vi "RTShutdown.vi"(0 "FPGA VI Reference In":refnum<k20>, 3 "error in (no error)":errorcluster) -> (10 "error out":errorcluster)   [LabVIEW 2016]
uses:
  <vilib>/Utility/error.llb/Error Cluster From Error Code.vi
  <vilib>/rvi/errors/niLvFpgaAdjustHostInterfaceError.vi
  <vilib>/FPGAPlugInAG/Dynamic/niLvFpga_Close_Dynamic.vi
  <vilib>/rvi/interface/nirviMethod/nirviMethod.xnode
  <vilib>/rvi/interface/nirviCloseFPGA/nirviCloseFPGA.xnode
  <vilib>/FPGAPlugInAG/Dynamic/niLvFpga_WriteFifo_Dynamic.vi
  <vilib>/rvi/errors/niLvFpgaMergeErrorWithErrorCode.vi
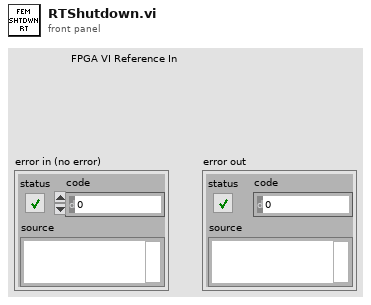
[diagram p1: front panel]
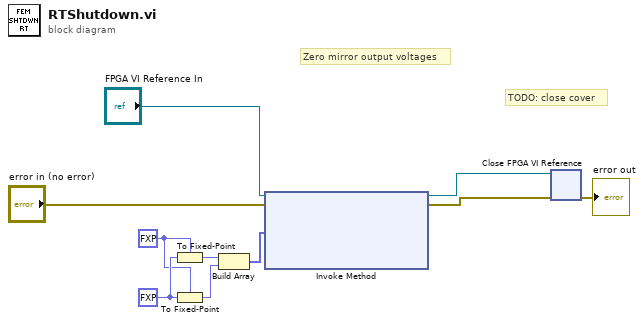
[diagram p0: block diagram]
diagram:
  w4 = fxp<+/-,32,16> 0.0 ("number")
  w1 = fxp<+/-,20,5> 0.0 ("fixed-point type")
  # "TODO: close cover"
  # "Zero mirror output voltages"
  n1 = To Fixed-Point(fixed-point type=w1, number=w4) -> (fixed-point=w5:fxp<+/-,20,5>)
  n2 = To Fixed-Point(fixed-point type=w1, number=w4) -> (fixed-point=w2:fxp<+/-,20,5>)
  n3 = Build Array(w5, w2) -> (w3:fxp<+/-,20,5>[])
  n4 = xnode "Invoke Method"("FPGA VI Reference In"="FPGA VI Reference In", "error in"="error in (no error)", "Data"=w3) -> ("FPGA VI Reference Out"=w6:refnum<k20>, "error out"=w8:errorcluster)  [unwired: 1 in, 1 out]
  n5 = xnode "Close FPGA VI Reference"("FPGA VI Reference In"=w6, "error in"=w8) -> ("error out"=→"error out":errorcluster)
